vi "MIDI-File_Loader.vi"(8 "Error In":errorcluster, 11 "MIDI-Data In":T2) -> (0 "Error Out":errorcluster, 3 "MIDI-Data Out":T2)   [LabVIEW 2019]
doc: "Loads text-files from midi_messages folder, compiles and populates MIDI-Message_Array."
uses:
  Controls/MIDI-Data.ctl
  Controls/MIDI-Message_Array.ctl
  Controls/MIDI-Message_Cluster.ctl
  Controls/Meta_Commands.ctl
  Common/Controls/Application_Message.ctl
  Common/Controls/Application_State.ctl
  <vilib>/Utility/error.llb/DialogType.ctl
panel:
  in  "Control Tab":T1(tab)
  out "Console Log":string
  out "Textfiles in midi_messages folder":string[](array[string])
  out "Error Message":string
  out "VI-filename":string
  out "VI Path":path
  out "Code Size":u32
  out "Revision Number":u32
  in  "Tool Bar:Visible":bool
  in  "Execution:Show Front Panel On Call":bool
  out "VI-Name":string
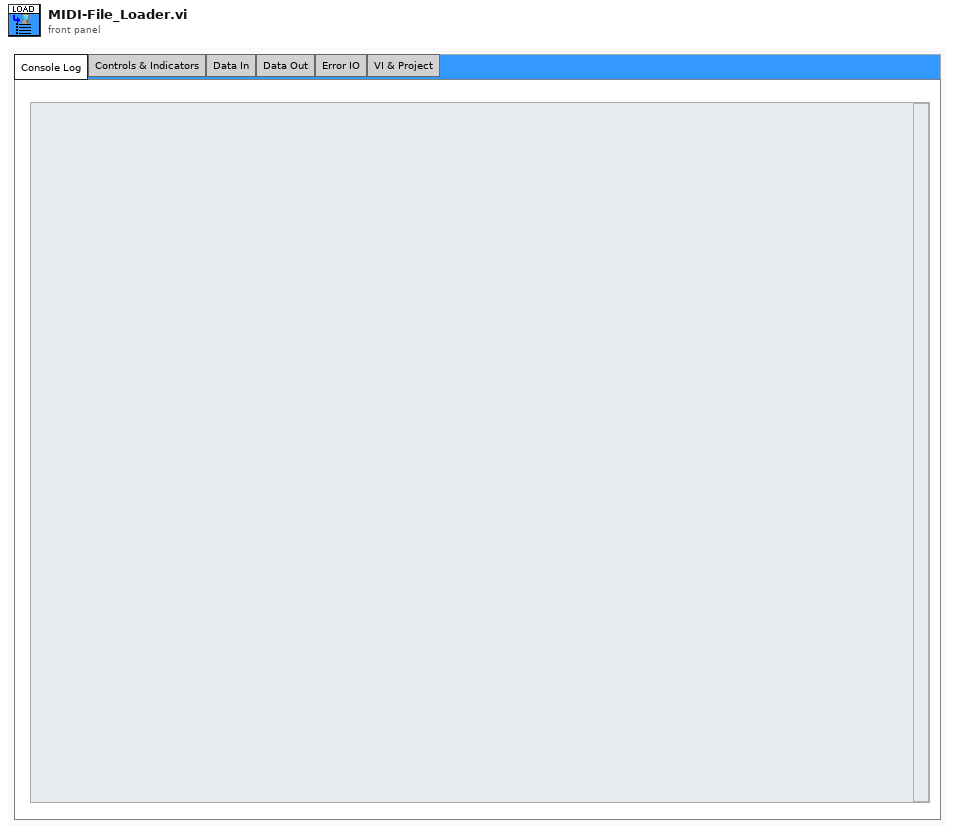
[diagram p1: front panel]
types:
  T1 = enum32{"Console Log", "Controls & Indicators", "Data In", "Data Out", "Error IO", "VI & Project"}
  T2 = typedef "MIDI-Data.ctl" = cluster{"Console log":string, "Payload":variant, "MIDI Message Array":T3, "Timout-Time[ms]":i32, "Queue_MIDI_Handler":refnum<queue>, "To_GUI-Error_message":refnum<user-event>, "To_GUI-msg_list":refnum<user-event>, "CPU(ms)":u32}
  T3 = typedef "MIDI-Message_Array.ctl" = T4[]
  T4 = typedef "MIDI-Message_Cluster.ctl" = cluster{"Message Name":string, "Meta value":i32, "Datastring":string, "Datatype":T5}
  T5 = typedef "Meta_Commands.ctl" = enum16{"No Data", "Pause", "Loop", "Wait for Rx", "Delay", "Break", "MIDI"}
  T6 = typedef "DialogType.ctl" = u16
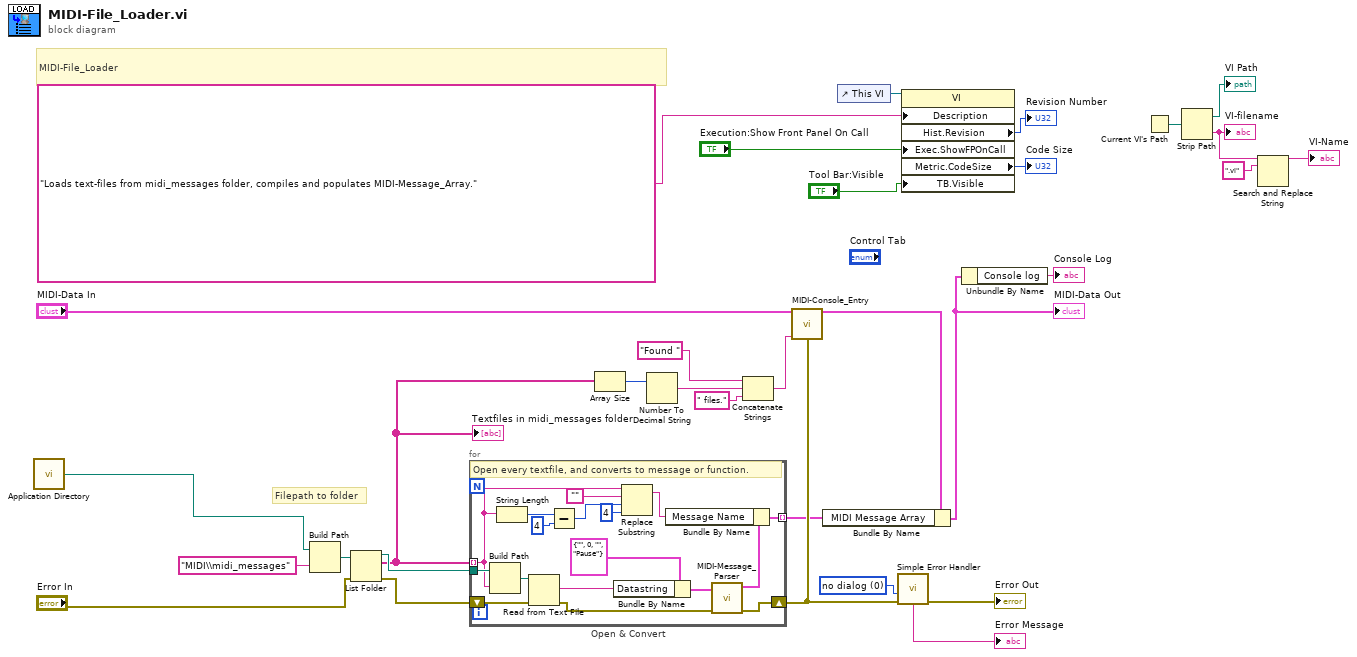
[diagram p0: block diagram]
diagram:
  w18 = T6 0 items=["no dialog", "OK message", "continue or stop message", "OK message + warnings", "continue/stop + warnings"] ("type of dialog (OK msg:1)")
  # "Filepath to folder"
  # "MIDI-File_Loader"
  n1 = call <vilib>:"Application Directory.vi"() -> ("Application Directory"=w4:path)
  n2 = Build Path(base path=w4, name or relative path="MIDI\\midi_messages") -> (appended path=w3:path)
  n3 = List Folder(path=w3, error in="Error In") -> (path out=w13:path, filenames=w2:string[], error out=w14:errorcluster)  [unwired: 2 in, 1 out]
  "Textfiles in midi_messages folder" <- w2
  n4 = for "Open & Convert" {
    tunnel: w2 -> [w45] mode=indexing
    tunnel: w13 -> [w49]
    shift-right: [w36] -> w6
    shift-left: w14 -> [w46]
    tunnel: [w43] -> w5 mode=indexing
    # "Open every textfile, and converts to message or function."
    n5 = Build Path(base path=w49, name or relative path=w45) -> (appended path=w47:path)
    n6 = String Length(string=w45) -> (length=w44:i32)
    n7 = Read from Text File(file (use dialog)=w47, error in=w46) -> (text=w33:string, error out=w37:errorcluster)  [unwired: 2 in, 2 out]
    n8 = Subtract(x=w44, y=4) -> (x-y=w39:i32)
    n9 = Bundle By Name(cluster=T4 {"Message Name"="", "Meta value"=0, "Datastring"="", "Datatype"=enum."Pause"} ("MIDI Message Cluster"), "Datastring"=w33) -> (w34:T4)
    n10 = Replace Substring(2:4 ("length (len. of substring)"), 3:w39, 4:"" ("substring (\"\")"), 5:w45) -> (1:w42:string)  [unwired: 1 out]
    n11 = call "MIDI-Message_Parser.vi"("Error In"=w37, "MIDI Message Cluster In"=w34) -> ("Error Out"=w36:errorcluster, "MIDI Message Cluster Out"=w41:T4)  [unwired: 8 in]
    n12 = Bundle By Name(cluster=w41, "Message Name"=w42) -> (w43:T4)
  }
  n13 = Array Size(array=w2) -> (size(s)=w12:i32)
  n14 = Number To Decimal String(number=w12) -> (decimal integer string=w11:string)  [unwired: 1 in]
  n15 = Concatenate Strings("Found " ("string"), w11, " files." ("string")) -> (w7:string)
  n16 = call "MIDI-Console_Entry.vi"("Data In"="MIDI-Data In", "Console Entry"=w7, "Error In"=w6) -> ("Data Out"=w8:T2)  [unwired: 12 in]
  n17 = Bundle By Name(cluster=w8, "MIDI Message Array"=w5) -> (w10:T2)
  "MIDI-Data Out" <- w10
  n18 = control-ref of="This VI"() -> (w26:refnum<vi>)
  n19 = call <vilib>:"Simple Error Handler.vi"("type of dialog (OK msg:1)"=w18, "error in (no error)"=w6) -> ("error out"=→"Error Out":errorcluster, "message"=→"Error Message":string)  [unwired: 3 in, 3 out]
  n20 = property class="VI"(reference=w26, "Description"="Loads text-files from midi_messages folder, compiles and populates MIDI-Message_Array.", "Exec.ShowFPOnCall"="Execution:Show Front Panel On Call", "TB.Visible"="Tool Bar:Visible") -> ("Hist.Revision"=→"Revision Number":u32, "Metric.CodeSize"=→"Code Size":u32)  [unwired: 1 in, 2 out]
  n21 = Unbundle By Name(w10) -> ("Console log"=→"Console Log":string)
  n22 = Current VI's Path() -> (path=w32:path)
  n23 = Strip Path(path=w32) -> (stripped path=→"VI Path":path, name=w23:string)
  "VI-filename" <- w23
  n24 = Search and Replace String(input string=w23, search string=".vi") -> (result string=→"VI-Name":string)  [unwired: 6 in, 3 out]
